vi "DOE Kitchen Data Agilent Compile.vi"(4 "Water Pressure":dbl, 5 "TC Coefficients":T2, 6 "Water Temperature":dbl, 7 "Agilent Digital Events":bool[](array[boolean]), 8 "Error In":errorcluster, 9 "Flow Rate":dbl, 10 "Data Logger Type":T1=enum."Agilent", 11 "Data Input":dbl[](array[numeric])) -> (0 "Error Out":errorcluster, 2 "Kitchen Analog Data":string[][](array[string]), 3 "Kitchen Cluster":T3)   [LabVIEW 2019]
uses:
  Type Definitions/DOE Kitchen Control.ctl
  Utility/Type Definitions/UTILITY TC Coefficients.ctl
  Type Definitions/DOE Data Logger Type.ctl
panel:
  out "Events":i32[](array[numeric])
  out "Spare":i32[](array[numeric])
  out "P and T":i32[](array[numeric])
  out "TC":i32[](array[numeric])
  out "sorted array":i32[](array[numeric])
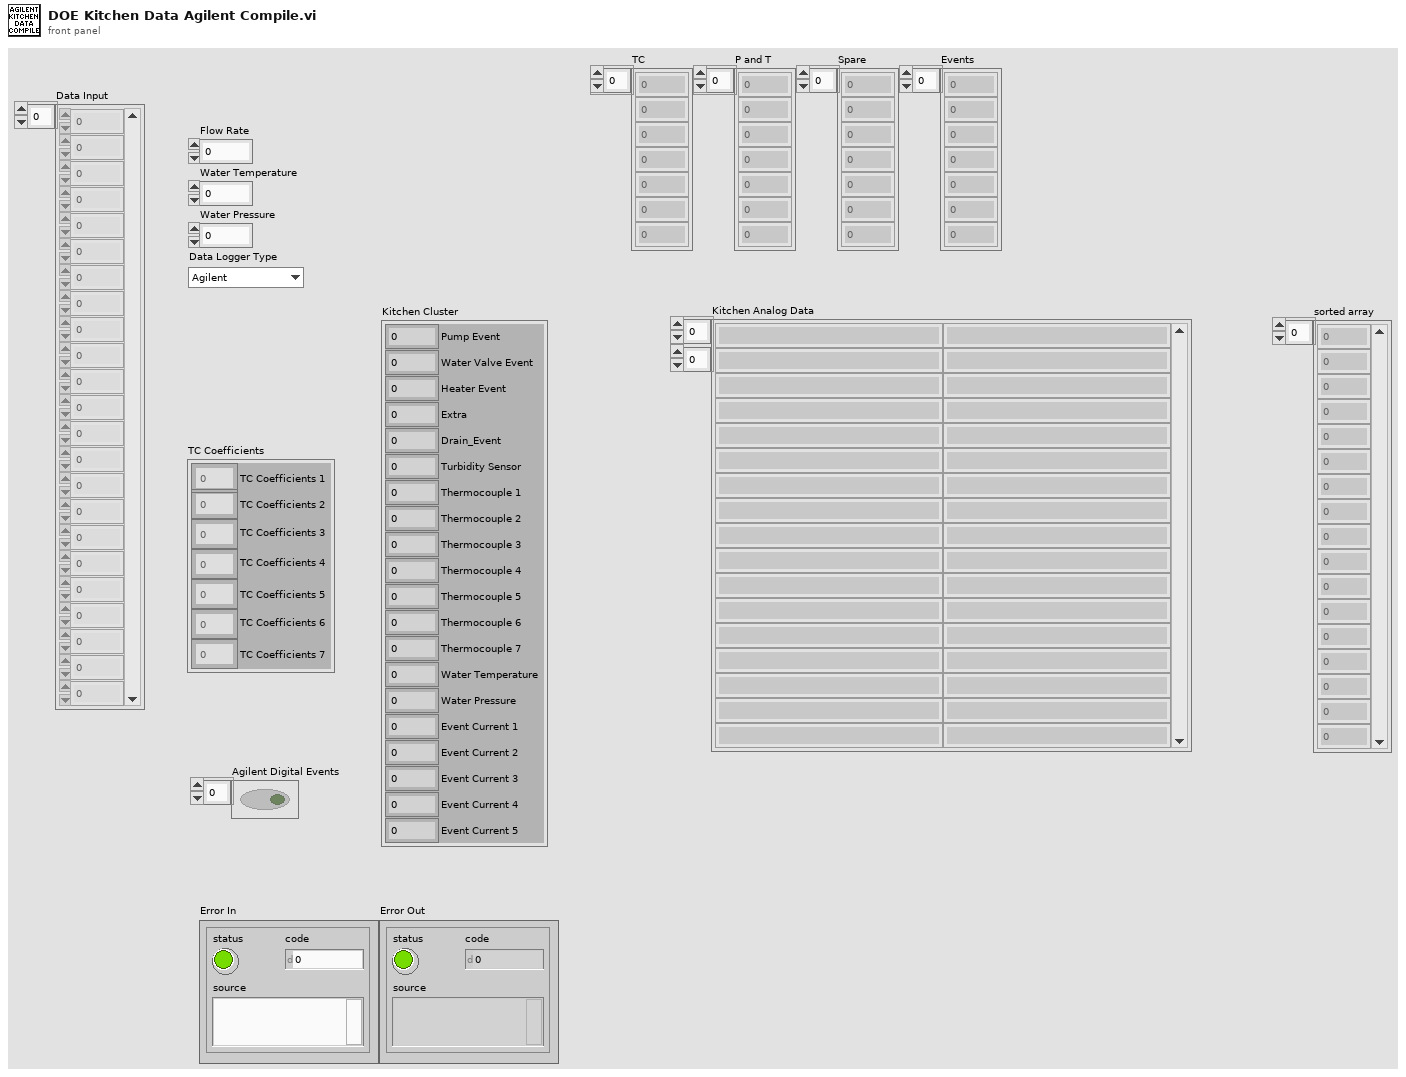
[diagram p1: front panel]
types:
  T1 = typedef "DOE Data Logger Type.ctl" = enum16{"MW100", "Agilent", "Agilent_Laurel_DC_Clamp"}
  T2 = typedef "UTILITY TC Coefficients.ctl" = cluster{"TC Coefficients 1":dbl[], "TC Coefficients 2":dbl[], "TC Coefficients 3":dbl[], "TC Coefficients 4":dbl[], "TC Coefficients 5":dbl[], "TC Coefficients 6":dbl[], "TC Coefficients 7":dbl[]}
  T3 = typedef "DOE Kitchen Control.ctl" = cluster{"Drain_Event":i16, "Pump Event":i16, "Water Valve Event":i16, "Heater Event":i16, "Extra":i16, "Turbidity Sensor":dbl, "Thermocouple 1":dbl, "Thermocouple 2":dbl, "Thermocouple 3":dbl, "Thermocouple 4":dbl, "Thermocouple 5":dbl, "Thermocouple 6":dbl, "Water Temperature":dbl, "Water Pressure":dbl, "Event Current 1":dbl, "Event Current 2":dbl, "Event Current 3":dbl, "Event Current 4":dbl, "Event Current 5":dbl, "Thermocouple 7":dbl}
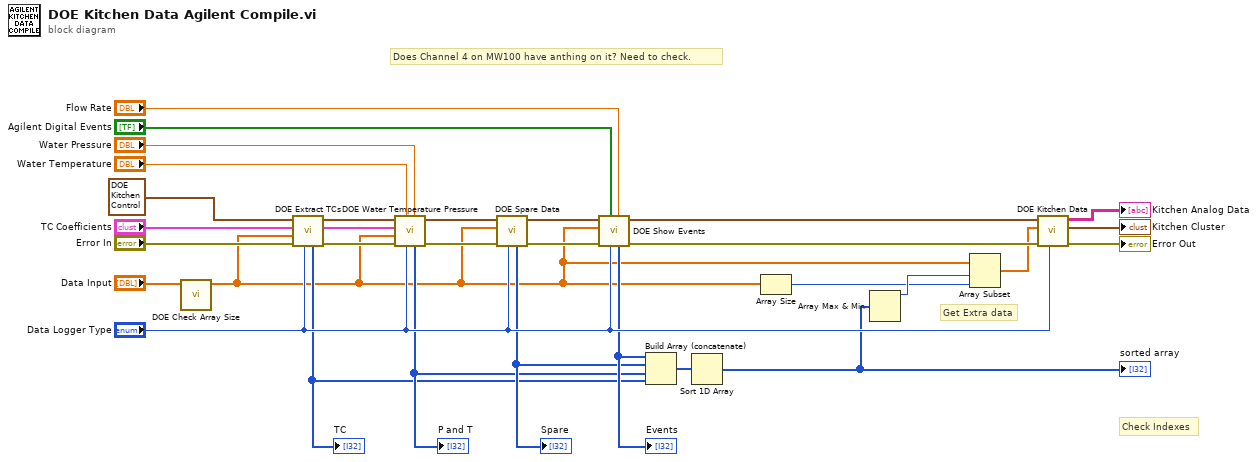
[diagram p0: block diagram]
diagram:
  # "Get Extra data"
  # "Check Indexes"
  # "Does Channel 4 on MW100 have anthing on it? Need to check."
  n1 = call "DOE Check Array Size.vi"("Data List"="Data Input") -> ("Output Array"=w4:dbl[])  [unwired: 9 in, 1 out]
  n2 = call "DOE Extract TCs.vi"("Data Logger Type"="Data Logger Type", "Error In"="Error In", "Agilent Array"=w4, "TC Coefficients"="TC Coefficients", "Kitchen Cluster in"=T3 {"Drain_Event"=0, "Pump Event"=0, "Water Valve Event"=0, "Heater Event"=0, "Extra"=0, "Turbidity Sensor"=0.0, "Thermocouple 1"=0.0, "Thermocouple 2"=0.0, "Thermocouple 3"=0.0, "Thermocouple 4"=0.0, "Thermocouple 5"=0.0, "Thermocouple 6"=0.0, "Water Temperature"=0.0, "Water Pressure"=0.0, "Event Current 1"=0.0, "Event Current 2"=0.0, "Event Current 3"=0.0, "Event Current 4"=0.0, "Event Current 5"=0.0, "Thermocouple 7"=0.0}) -> ("Error Out"=w21:errorcluster, "TC Coefficients Out"=w20:T2, "Kitchen Cluster out"=w23:T3, "appended array"=w8:i32[])  [unwired: 3 in]
  "TC" <- w8
  n3 = call "DOE Water Temperature Pressure.vi"("Water Pressure"="Water Pressure", "Data Logger Type"="Data Logger Type", "Water Temperature"="Water Temperature", "Error In"=w21, "Output Array"=w4, "TC Coefficients"=w20, "Kitchen Cluster in"=w23) -> ("Error Out"=w19:errorcluster, "Kitchen Cluster out"=w22:T3, "sorted array"=w9:i32[])  [unwired: 2 in]
  "P and T" <- w9
  n4 = call "DOE Spare Data.vi"("Data Logger Type"="Data Logger Type", "Error In"=w19, "Output Array"=w4, "Kitchen Cluster in"=w22) -> ("Error Out"=w16:errorcluster, "Kitchen Cluster out 2"=w17:T3, "sorted array"=w10:i32[])  [unwired: 5 in]
  "Spare" <- w10
  n5 = call "DOE Show Events.vi"("Flow Rate"="Flow Rate", "Data Logger Type"="Data Logger Type", "Agilent Digital Events"="Agilent Digital Events", "Error In"=w16, "Data Input"=w4, "Kitchen Cluster Inlet"=w17) -> ("Error Out"=w15:errorcluster, "Kitchen Cluster Output"=w24:T3, "sorted array"=w11:i32[])  [unwired: 3 in]
  "Events" <- w11
  n6 = Build Array (concatenate)(w11, w10, w9, w8) -> (w7:i32[])
  n7 = Sort 1D Array(array=w7) -> (sorted array=w6:i32[])
  "sorted array" <- w6
  n8 = Array Size(array=w4) -> (size(s)=w3:i32)
  n9 = Array Max & Min(array=w6) -> (max value=w5:i32)  [unwired: 3 out]
  n10 = Array Subset(array=w4, index=w5, length=w3) -> (w2:dbl[])
  n11 = call "DOE Kitchen Data.vi"("Data Logger Type"="Data Logger Type", "Error In"=w15, "Extra Data"=w2, "Kitchen Input"=w24) -> ("Error Out"=→"Error Out":errorcluster, "Kitchen Cluster"=→"Kitchen Cluster":T3, "Kitchen Analog Data"=→"Kitchen Analog Data":string[][])  [unwired: 4 in, 1 out]
